vi "SendMessages.vi"(4 "message values":string[](array[string]), 5 "message names":string[](array[string]), 6 "error in":errorcluster, 7 "timeout in ms (-1)":i32, 9 "message queue in":T1) -> (0 "error out":errorcluster, 1 "timed out":bool[](array[boolean]), 3 "message queue out":T1)   [LabVIEW 2014, in "SimpleMessaging.lvlib"]
uses:
  SimpleMessaging.lvlib
  MessageQueueTD.ctl
  MessageTD.ctl
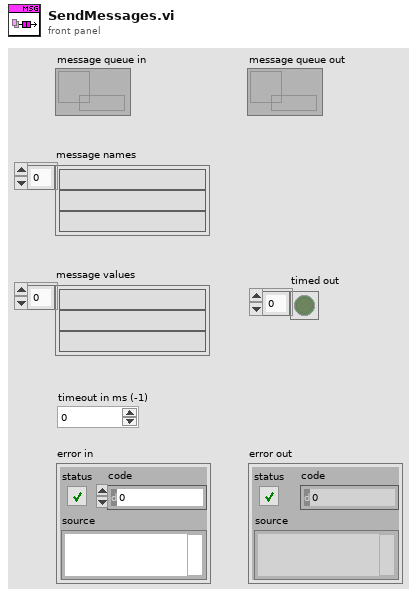
[diagram p1: front panel]
types:
  T1 = typedef "SimpleMessaging.lvlib/MessageQueueTD.ctl" = refnum<queue>
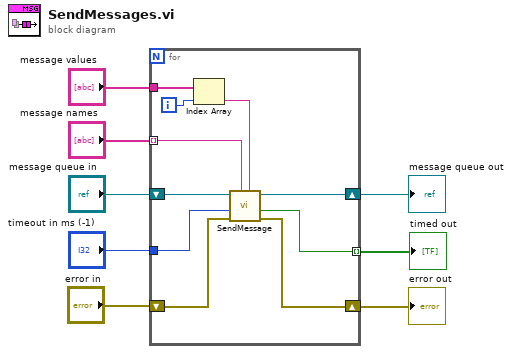
[diagram p0: block diagram]
diagram:
  n1 = for {
    shift-right: [w17] -> w7
    shift-left: "message queue in" -> [w18]
    tunnel: "message names" -> [w16] mode=indexing
    tunnel: "message values" -> [w11]
    tunnel: "timeout in ms (-1)" -> [w15]
    shift-right: [w12] -> w2
    shift-left: "error in" -> [w14]
    tunnel: [w13] -> w1 mode=indexing
    i -> [w9]
    n2 = Index Array(array=w11, index=w9) -> (element=w10:string)
    n3 = call "SendMessage.vi"("Value"=w10, "Name"=w16, "error in"=w14, "timeout in ms (-1)"=w15, "message queue in"=w18) -> ("error out"=w12:errorcluster, "timed out?"=w13:bool, "message queue out"=w17:T1)  [unwired: 2 in]
  }
  "message queue out" <- w7
  "error out" <- w2
  "timed out" <- w1
